vi "WriteCmd.vi"(2 "error IO":errorcluster, 3 "Command":string, 4 "VISA resource name":refnum<visa-resource-name>) -> (0 "error":errorcluster, 1 "VISA out":refnum<visa-resource-name>)   [LabVIEW 2018]
doc: "This VI flushes the transmit buffer and transmits a command.\nNote that the input command need not contain CR LF because those characters are concatenated onto the input string.\nNote that 40, the integer argument for VISA Flush I/O Buffer,s is hexadecimal."
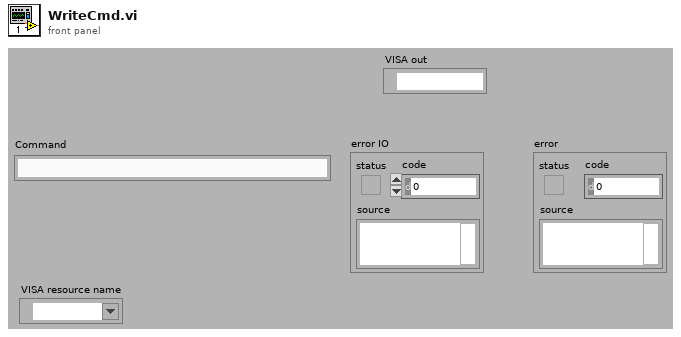
[diagram p1: front panel]
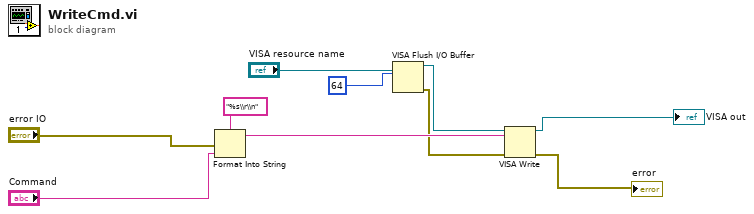
[diagram p0: block diagram]
diagram:
  n1 = Format Into String "Format Into String"(format string="%s\\r\\n", error in="error IO", "Command") -> (resulting string=w8:string)  [unwired: 1 in, 1 out]
  n2 = VISA Flush I/O Buffer(VISA resource name="VISA resource name", mask (16)=u16 64) -> (VISA resource name out=w4:refnum<visa-resource-name>, error out=w3:errorcluster)  [unwired: 1 in]
  n3 = VISA Write(VISA resource name=w4, write buffer=w8, error in (no error)=w3) -> (VISA resource name out=→"VISA out":refnum<visa-resource-name>, error out=→"error":errorcluster)  [unwired: 1 out]
